vi "Publish FC1 ILC Inputs.vi"(8 "error in (no error)":errorcluster, 11 "Model in":refnum<class "Model.lvclass">) -> (0 "error out":errorcluster, 3 "Model out":refnum<class "Model.lvclass">)   [LabVIEW 2015, in "Model.lvclass"]
uses:
  Model.lvclass
  Model.lvclass/Model.ctl
  <userlib>/Common/ILC/ILC/ILC.lvclass/ILC.ctl
  User Events/User Events.lvclass/User Events.ctl
  User Events/User Events.lvclass
  <userlib>/Common/ILC/ILC/ILC.lvclass
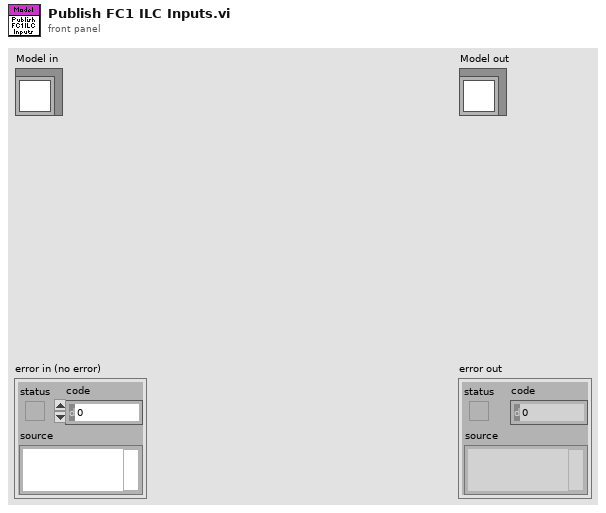
[diagram p1: front panel]
types:
  T1 = typedef "ILCCommon.lvlib/ILCTypedefs.lvlib/ADC Eng.ctl" = cluster{"Ch1":dbl[unit], "Ch2":dbl[unit], "Ch3":dbl[unit], "Ch4":dbl[unit]}
  T2 = typedef "FAMT Typedefs.lvlib/Publish Data Events.ctl" = cluster{"State":refnum<user-event>, "ErrorCode":refnum<user-event>, "FC1 ILC Outputs":refnum<user-event>, "LogPath":refnum<user-event>, "FC1 ILC Inputs":refnum<user-event>, "Scan Progress":refnum<user-event>, "FC2 ILC Outputs":refnum<user-event>, "FC2 ILC Inputs":refnum<user-event>}
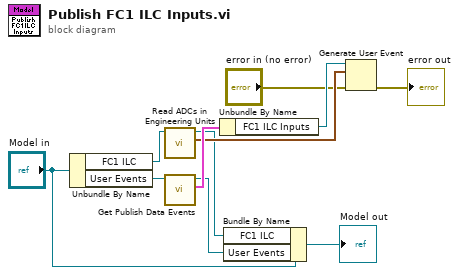
[diagram p0: block diagram]
diagram:
  n1 = Unbundle By Name("Model in") -> ("FC1 ILC"=w10:refnum<class "ILC.lvclass">, "User Events"=w5:refnum<class "User Events.lvclass">)
  n2 = call <userlib>:"Read ADCs in Engineering Units.vi"("ILC in"=w10) -> ("ADCs in Engineering Units"=w6:T1, "ILC out"=w3:refnum<class "ILC.lvclass">)  [unwired: 9 in]
  n3 = call "Get Publish Data Events.vi"("UserEvents in"=w5) -> ("Publish Data Events"=w11:T2, "UserEvents out"=w4:refnum<class "User Events.lvclass">)  [unwired: 9 in]
  n4 = Unbundle By Name(w11) -> ("FC1 ILC Inputs"=w9:refnum<user-event>)
  n5 = Bundle By Name(cluster="Model in", "FC1 ILC"=w3, "User Events"=w4) -> (→"Model out":refnum<class "Model.lvclass">)
  n6 = Generate User Event(user event=w9, event data cluster=w6, error in="error in (no error)") -> (error out=→"error out":errorcluster)  [unwired: 1 in, 1 out]
